vi "cornell-plot.vi"() -> ()   [LabVIEW 2020]
uses:
  cornell-Ktildesh2sides.ctl
  cursor action.ctl
  2Dwindow.ctl
  array action.ctl
  16981a69-1a1c-c642-ac20-7ef28ecb8088.vi
  replace cursor action stack.vi
  Q -- range multiplier -- real -- V2.vi
  Q - not nan and gtr than zero - Real.vi
  Q - not nan -- real.vi
  Q -- check range -- i -- real.vi
  array - smart min max.vi
  cornell-K0edges.vi
  cornell-K0s.vi
  <vilib>/Comparison/Less/Less Functor/Less Functor.lvclass
panel:
  in  "everything I need to know about heat conductivity and I mean everything":T1(tab)
  in  "parameter selectors":enum32{"Page 1"}(tab)
  in  "scale gauge: Plot: complex plane":dbl(slide)=6.232708 min=0.0 max=0.3 step=1e-06 scale=0.01..100000.0 scale format="%#_3p"
  out "Plot: sweep window":cluster{"Freq out (Hz)":dbl[], dbl[]}[](graph)
  out "Ktilde":cdb=0.005910268621655171+0.3162087805454639i format="%#_2p"
  in  "what to plot":T2=enum."plot: two½"
  in  "ω0 (rad/sec)":dbl(slide)=6.660846290809155 scale=0.001..10000.0 scale format="%#_2p"
  in  "parameter selectors 3":enum32{"Page 1"}(tab)
  out "Plot: vs s":cluster{dbl[], dbl[]}[](graph)
  in  "scale gauge: Plot: vs s":dbl(slide)=0.5231559999999998 min=0.0 max=0.3 step=1e-06 scale=0.01..10.0 scale format="%#_3p"
  in  "sample pars":T3={"τR (sec)"=0.154639, "L2DS (sec)"=3.81679389313, "τL (sec)"=10.0, "s/L"=0.0, "h/L"=0.22900799999999996} {"h/L" min=0.0 max=0.3 step=1e-06 scale=0.0..1.0 scale format="%#_3p"; "s/L" min=0.0 max=0.3 step=1e-06 scale=0.0..1.0 scale format="%#_3p"; "τL (sec)" min=0.0 max=0.3 step=1e-06 scale=0.0..100.0 scale format="%#_3p"; "L2DS (sec)" min=0.0 max=0.3 step=1e-12 scale=0.001..10.0 scale format="%#_3p"; "τR (sec)" min=0.0 max=0.3 step=1e-06 scale=0.0..100.0 scale format="%#_3p"}
  in  "plot pars":T4={"# of terms in the series"=500, "# plot points"=738, "min ω (rad/sec)"=0.0009999999999999994, "max ω (rad/sec)"=10000.00000000001} {"max ω (rad/sec)" scale=0.001..5000.0; "min ω (rad/sec)" scale=0.001..5000.0; "# plot points" scale=0.001..1500.0; "# of terms in the series" scale=0.001..1000.0}
  in  "cal pars":T5={"τS (sec)"=0.611076335878, "τC (sec)"=0.039129770992, " ζ"=0.818625954198, "κ0"=1.0} {"κ0" min=0.0 max=0.3 step=1e-12 scale=1e-10..1e-07 scale format="%#_3p"; "ζ" min=0.0 max=0.3 step=1e-12 scale=0.01..1.0 scale format="%#_3p"; "τC (sec)" min=0.0 max=0.3 step=1e-12 scale=0.001..1.0 scale format="%#_3p"; "τS (sec)" min=0.0 max=0.3 step=1e-12 scale=0.001..1.0 scale format="%#_3p"}
  in  "pause!":bool
  in  "go!":bool
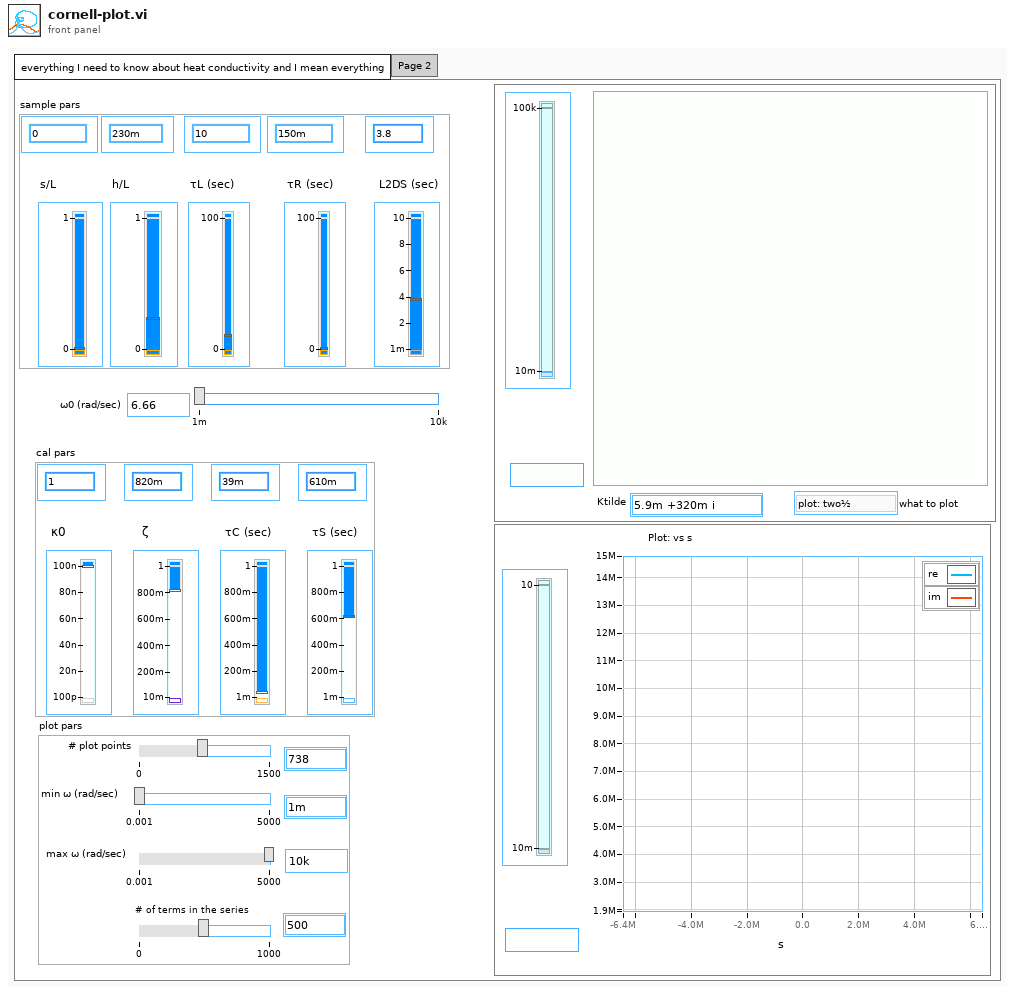
[diagram p1: front panel]
types:
  T1 = enum32{"everything I need to know about heat conductivity and I mean everything", "Page 2"}
  T2 = typedef "cornell-Ktildesh2sides.ctl" = enum16{"plot: check1", "plot: check2", "plot: one½", "plot: two½", "plot: uni½", "calc: zcoth(z)", "calc: z/sinh(z)", "calc: brute", "calc: integra", "void", "plot: nano"}
  T3 = cluster{"τR (sec)":dbl, "L2DS (sec)":dbl, "τL (sec)":dbl, "s/L":dbl, "h/L":dbl}
  T4 = cluster{"# of terms in the series":i64, "# plot points":i64, "min ω (rad/sec)":dbl, "max ω (rad/sec)":dbl}
  T5 = cluster{"τS (sec)":dbl, "τC (sec)":dbl, " ζ":dbl, "κ0":dbl}
  T6 = typedef "2Dwindow.ctl" = cluster{"window y":dbl, "center x":dbl, "center y":dbl, "window x":dbl}
  T7 = typedef "cursor action.ctl" = enum16{"range", "read", "write", "check", "zoom out", "smart zoom out", "zoom to aspect ratio 1", "zoom to win", "zoom out 20%", "zoom in 20%", "-empty", "smart zoom out&aspect", "move range left 20%", "move range right 20%", "move range up 20%", "move range down 20%", "zoom to X win", "zoom to Y win", "zoom out X", "zoom out Y", "zoom in X", "zoom in Y", "check plot scale", "set plot color", "set Xlabel", "set Ylabel", "set cursor color"}
  T8 = typedef "array action.ctl" = enum16{"generate range", "generate log range"}
  T9 = typedef "eventvkey.ctl" = enum16{"ASCII", "Enter", "Return", "Shift", "Ctrl", "Alt", "Cmd", "Opt", "Caps", "NumLock", "Clear", "Break", "Up", "Down", "Left", "Right", "Insert", "Delete", "Home", "End", "PageUp", "PageDown", "Escape", "Help", "Pause", "ScrollLock", "F1", "F2", "F3", "F4", "F5", "F6", "F7", "F8", "F9", "F10", "F11", "F12", "F13", "F14", "F15", "F16", "F17", "F18", "F19", "F20", "F21", "F22", "F23", "F24", "Play", "VolumeUp", "VolumeDown", "Mute", "Two Byte Char"}
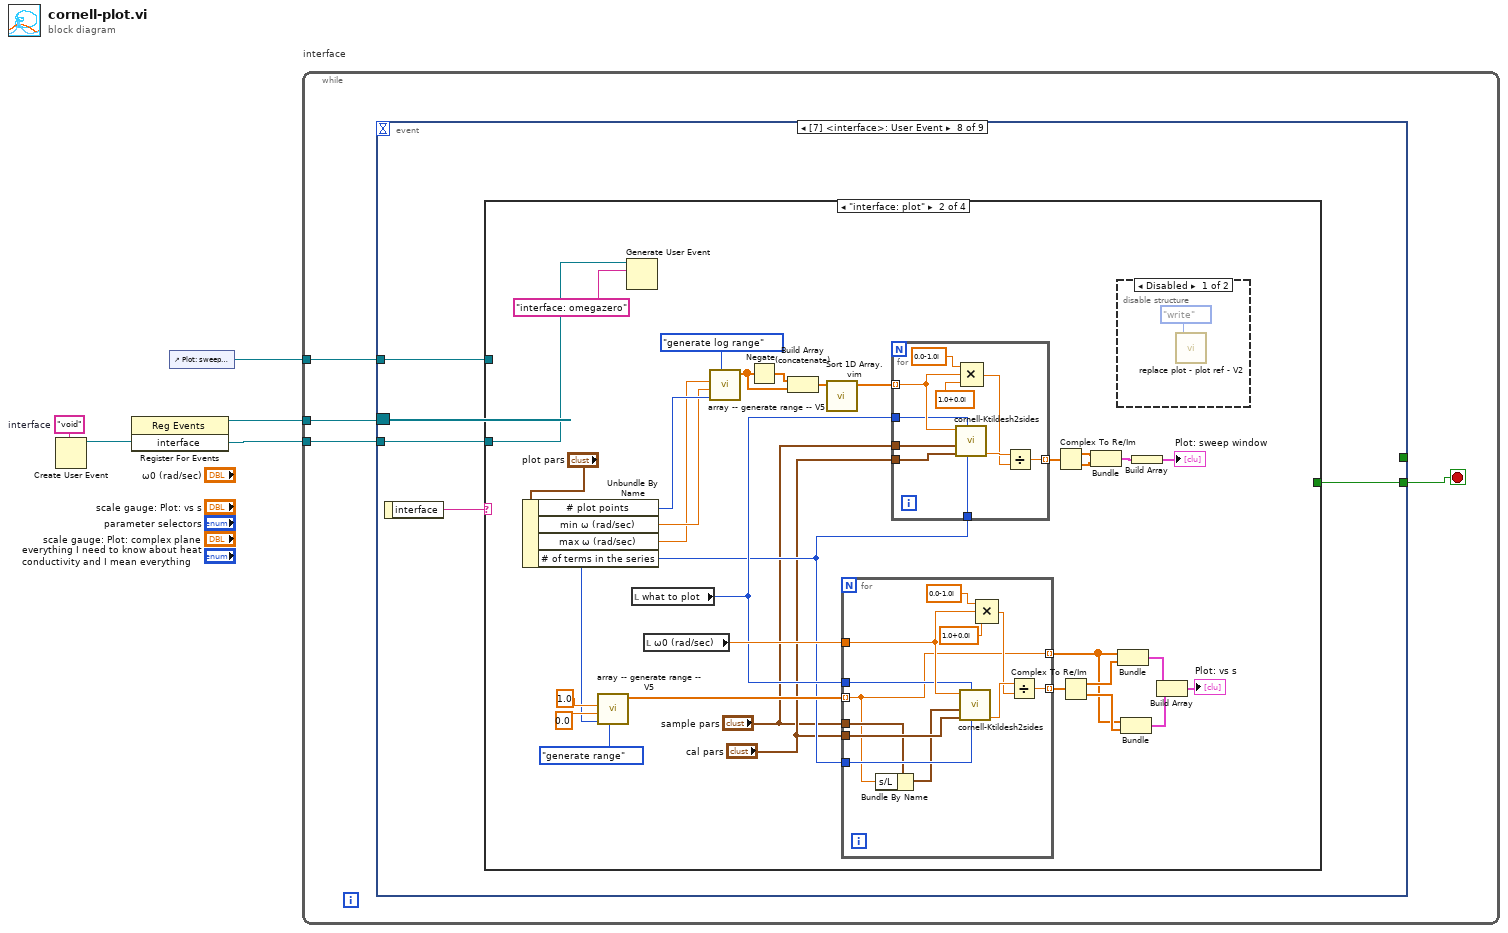
[diagram p0: block diagram]
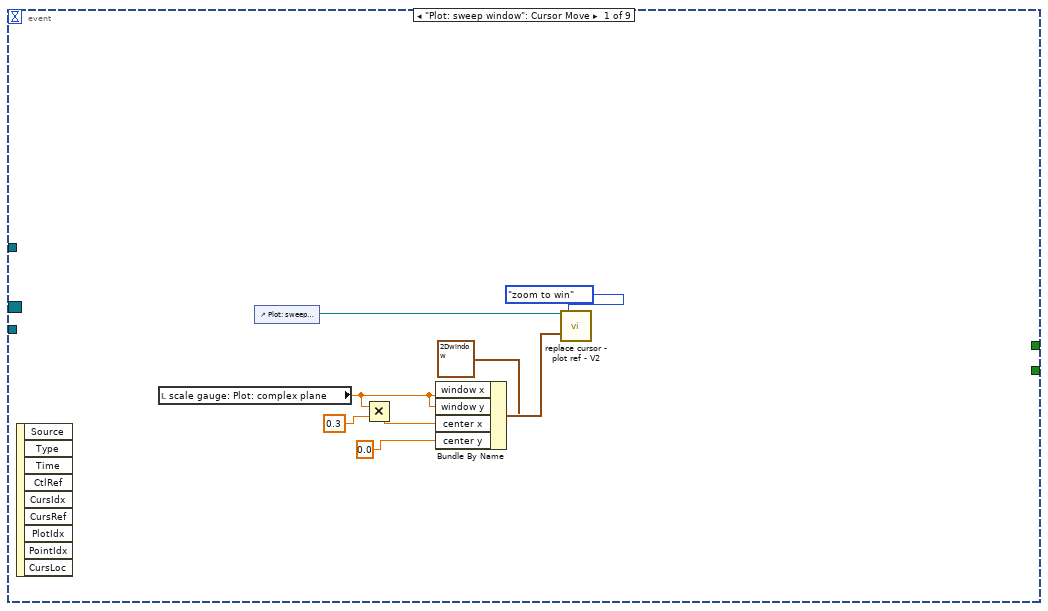
[diagram p2: hidden frame]
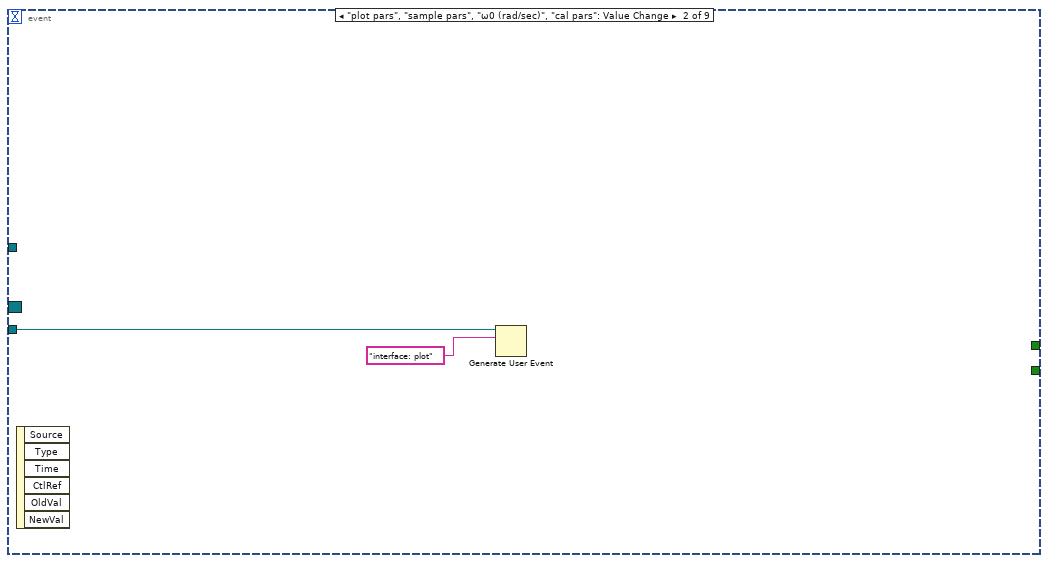
[diagram p3: hidden frame]
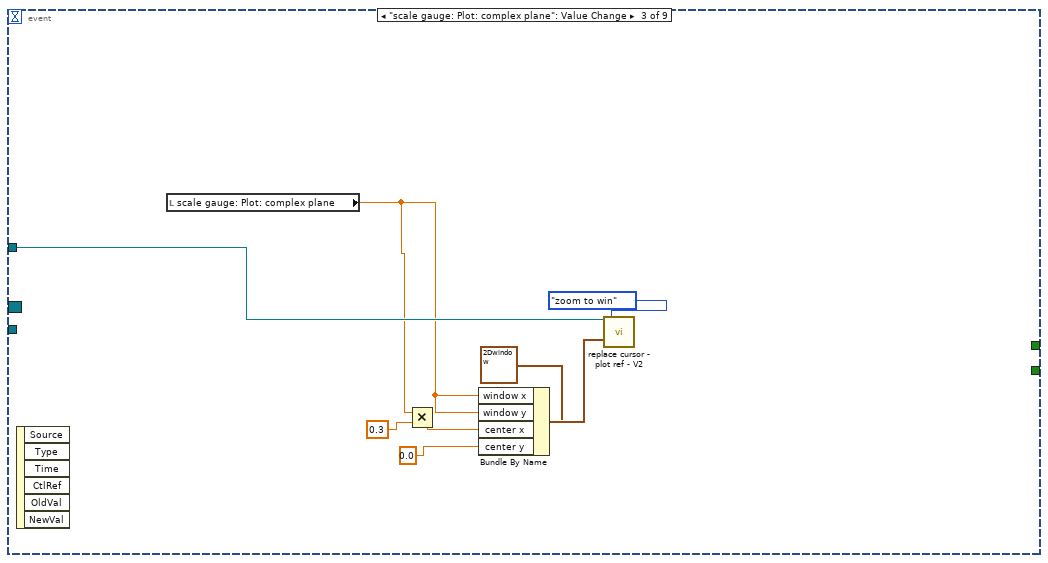
[diagram p4: hidden frame]
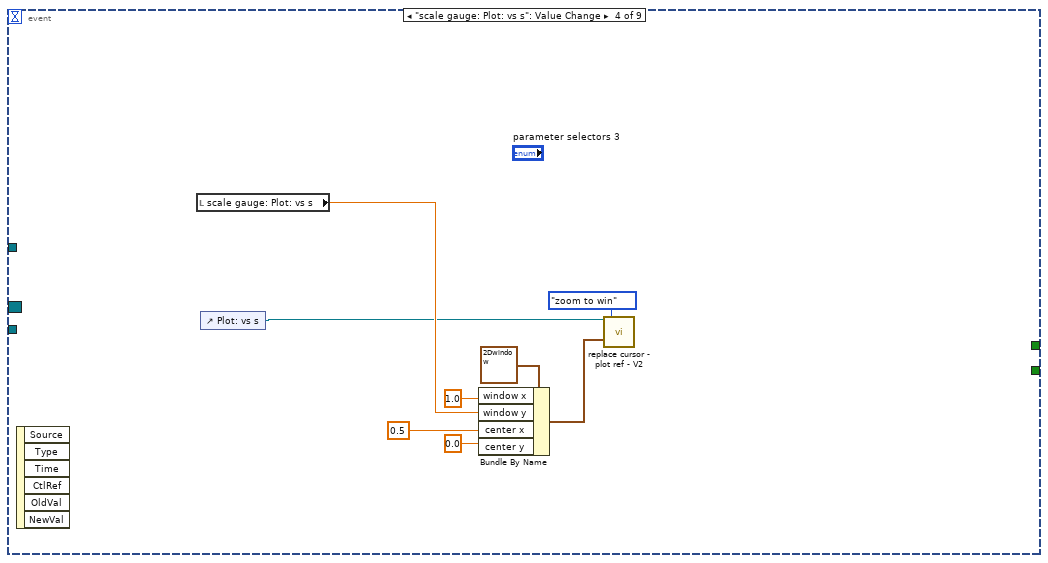
[diagram p5: hidden frame]
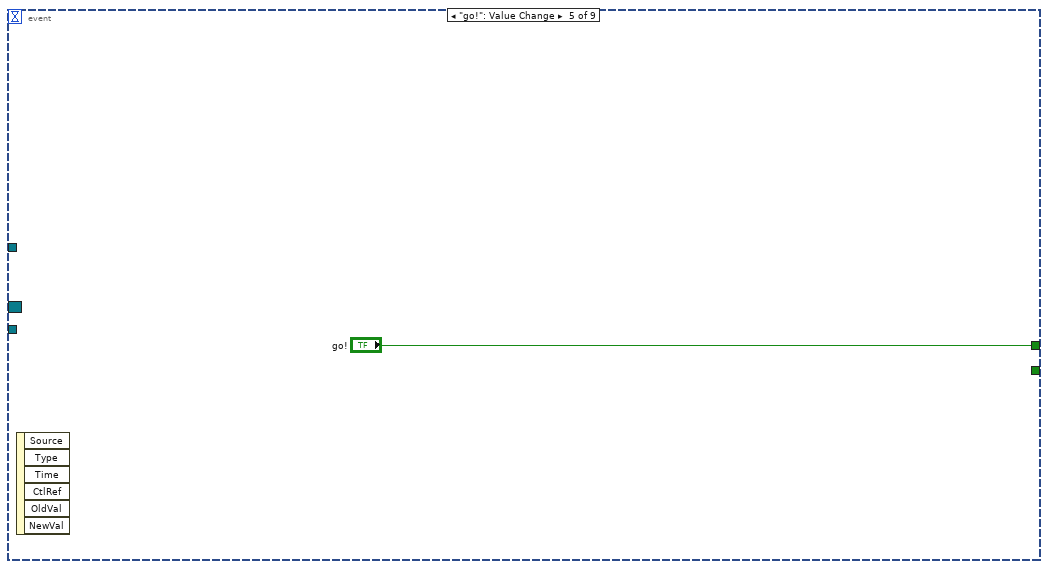
[diagram p6: hidden frame]
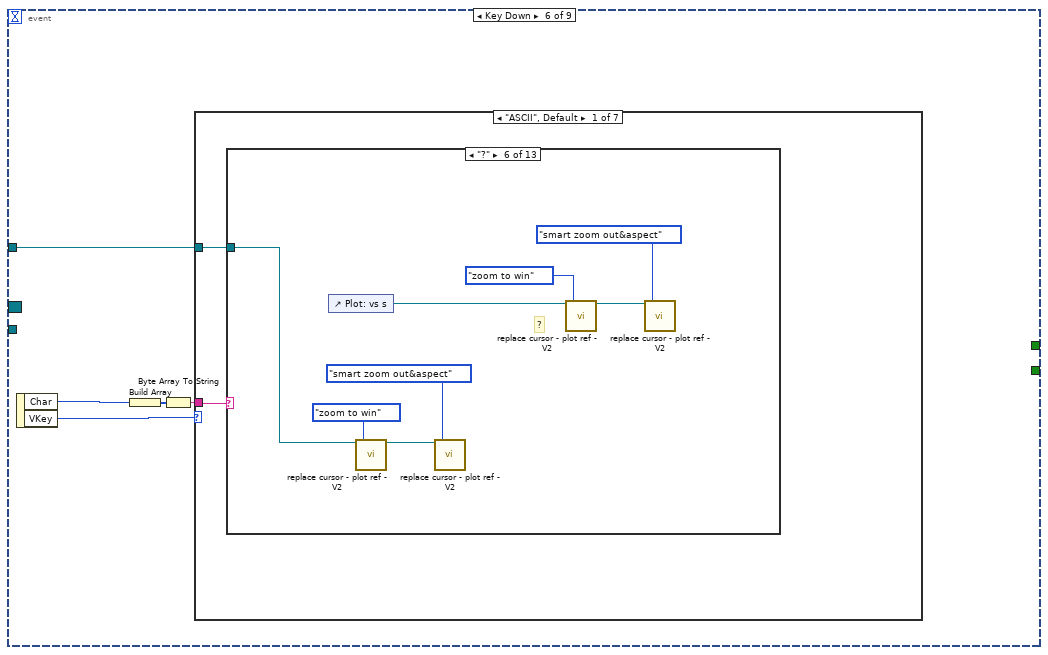
[diagram p7: hidden frame]
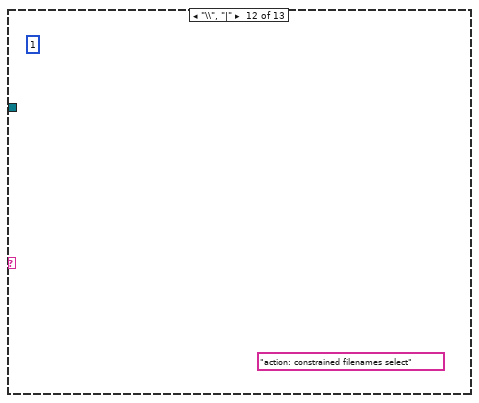
[diagram p18: hidden frame]
diagram:
  w3 = "void"  # interface
  n1 = Create User Event(user event datatype=w3) -> (user event=w1:refnum<user-event>)  [unwired: 1 in, 1 out]
  n2 = register-events(w1) -> (reference out=w4:refnum<event-registration>)  [unwired: 2 in, 1 out]
  n3 = control-ref of="Plot: sweep window"() -> (w2:refnum<vi>)
  n4 = while "interface" {
    tunnel: w4 -> [w8]
    tunnel: w2 -> [w7]
    tunnel: w1 -> [w6]
    stop <- w5 stop-if-true
    n5 = event shown="[7] <interface>: User Event" {
      selector: w8 -> [_ _ _ _ _ _ _ _ _]
      dyn-events: _ -> [_ _ _ _ _ _ _ _ _]
      timeout: _ -> [_ _ _ _ _ _ _ _ _]
      tunnel: [_ _ _ _ "go!" _ "pause!" _ _] -> _
      tunnel: w7 -> [_ _ w20 _ _ w36 _ w60 _]
      tunnel: w6 -> [_ w17 _ _ _ _ _ w59 w138]
      tunnel: [_ _ _ _ _ _ _ w61 _] -> w5
      event "Plot: sweep window": Cursor Move {
        n6 = event-data() -> ()  [unwired: 1 in, 9 out]
        n7 = local read "scale gauge: Plot: complex plane"() -> (w15:dbl)
        n8 = control-ref of="Plot: sweep window"() -> (w14:refnum<vi>)
        n9 = Multiply(x=w15, y=0.3) -> (x*y=w16:dbl)
        n10 = Bundle By Name(cluster=T6 {"window y"=0.0021014740628288917, "center x"=44850.89441339177, "center y"=2.5658109925320947, "window x"=17480.201988350764} ("window IN"), "window x"=w15, "window y"=w15, "center x"=w16, "center y"=0.0) -> (w13:T6)
        n11 = call "replace cursor - plot ref - V2.vi"("Plot ref in"=w14, "window IN"=w13, "cursor action"=cursor_action."zoom to win") -> ()  [unwired: 13 in, 4 out]
      }
      event "plot pars", "sample pars", "ω0 (rad/sec)", "cal pars": Value Change {
        n12 = event-data() -> ()  [unwired: 1 in, 6 out]
        n13 = Generate User Event(user event=w17, event data cluster="interface: plot" ("event data")) -> ()  [unwired: 2 in, 2 out]
      }
      event "scale gauge: Plot: complex plane": Value Change {
        n14 = event-data() -> ()  [unwired: 1 in, 6 out]
        n15 = local read "scale gauge: Plot: complex plane"() -> (w19:dbl)
        n16 = Multiply(x=w19, y=0.3) -> (x*y=w26:dbl)
        n17 = Bundle By Name(cluster=T6 {"window y"=0.0021014740628288917, "center x"=44850.89441339177, "center y"=2.5658109925320947, "window x"=17480.201988350764} ("window IN"), "window x"=w19, "window y"=w19, "center x"=w26, "center y"=0.0) -> (w25:T6)
        n18 = call "replace cursor - plot ref - V2.vi"("Plot ref in"=w20, "window IN"=w25, "cursor action"=cursor_action."zoom to win") -> ()  [unwired: 13 in, 4 out]
      }
      event "scale gauge: Plot: vs s": Value Change {
        n19 = event-data() -> ()  [unwired: 1 in, 6 out]
        n20 = local read "scale gauge: Plot: vs s"() -> (w30:dbl)
        n21 = control-ref of="Plot: vs s"() -> (w29:refnum<vi>)
        n22 = Bundle By Name(cluster=T6 {"window y"=0.0021014740628288917, "center x"=44850.89441339177, "center y"=2.5658109925320947, "window x"=17480.201988350764} ("window IN"), "window x"=1.0, "window y"=w30, "center x"=0.5, "center y"=0.0) -> (w34:T6)
        n23 = call "replace cursor - plot ref - V2.vi"("Plot ref in"=w29, "window IN"=w34, "cursor action"=cursor_action."zoom to win") -> ()  [unwired: 13 in, 4 out]
      }
      event "go!": Value Change {
        n24 = event-data() -> ()  [unwired: 1 in, 6 out]
      }
      event Key Down {
        n25 = event-data() -> ("Char"=w38:i16, "VKey"=w40:T9)  [unwired: 1 in]
        n26 = Build Array(w38) -> (w39:i16[])
        n27 = Byte Array To String(unsigned byte array=w39) -> (string=w37:string)
        n28 = case shown="\"ASCII\", Default" w40 {
          selector: w40 -> [_ _ _ _ _ _ w52]
          tunnel: w37 -> [w42 _ _ _ _ _ _]
          tunnel: w36 -> [w41 _ _ _ _ _ w51]
          frame "ASCII", Default {
            n29 = case shown="\"?\"" w42 {
              tunnel: w41 -> [_ _ _ _ _ w47 _ _ _ _ _ _ _]
              frame "0", Default {
              }
              frame "a" {
              }
              frame "s" {
              }
              frame "l" {
              }
              frame " " {
              }
              frame "?" {
                # "?"
                n30 = control-ref of="Plot: vs s"() -> (w43:refnum<vi>)
                n31 = call "replace cursor - plot ref - V2.vi"("Plot ref in"=w47, "cursor action"=cursor_action."zoom to win") -> ("Plot ref out"=w50:refnum<vi>)  [unwired: 14 in, 3 out]
                n32 = call "replace cursor - plot ref - V2.vi"("Plot ref in"=w50, "cursor action"=cursor_action."smart zoom out&aspect") -> ()  [unwired: 14 in, 4 out]
                n33 = call "replace cursor - plot ref - V2.vi"("Plot ref in"=w43, "cursor action"=cursor_action."zoom to win") -> ("Plot ref out"=w46:refnum<vi>)  [unwired: 14 in, 3 out]
                n34 = call "replace cursor - plot ref - V2.vi"("Plot ref in"=w46, "cursor action"=cursor_action."smart zoom out&aspect") -> ()  [unwired: 14 in, 4 out]
              }
              frame "+", ",", "-", ".", "<", "=", ">" {
              }
              frame "b" {
              }
              frame "u" {
              }
              frame "p" {
              }
              frame "q" {
              }
              frame "\\", "|" {
                (unwired) 1
                (unwired) "action: constrained filenames select" ("event data")
              }
              frame "m" {
              }
            }
          }
          frame "Escape" {
          }
          frame "PageUp" {
          }
          frame "Enter" {
          }
          frame "Caps" {
          }
          frame "PageDown" {
          }
          frame "Up".."Right" {
            n35 = case shown="\"Down\"" w52 {
              tunnel: [cursor_action."zoom in 20%" ("cursor action") cursor_action."zoom out 20%" ("cursor action") cursor_action."zoom out 20%" ("cursor action") cursor_action."zoom in 20%" ("cursor action")] -> w53
              frame "Up", Default {
              }
              frame "Down" {
              }
              frame "Left" {
              }
              frame "Right" {
              }
            }
            n36 = call "replace cursor - plot ref - V2.vi"("Plot ref in"=w51, "cursor action"=w53) -> ()  [unwired: 14 in, 4 out]
          }
        }
      }
      event "pause!": Value Change {
        n37 = event-data() -> ()  [unwired: 1 in, 6 out]
      }
      event User Event {
        n38 = event-data() -> ("interface"=w62:string)  [unwired: 1 in]
        n39 = case shown="\"interface: plot\"" w62 {
          tunnel: [_ _ TRUE _] -> w61
          tunnel: w60 -> [_ _ _ w130]
          tunnel: w59 -> [_ w84 _ _]
          frame "void", Default {
          }
          frame "interface: plot" {
            n40 = Unbundle By Name("plot pars") -> ("# plot points"=w69:i64, "min ω (rad/sec)"=w67:dbl, "max ω (rad/sec)"=w66:dbl, "# of terms in the series"=w68:i64)
            n41 = call "array -- generate range -- V5.vi"("action"=array_action."generate range", "ω points"=w69, "ω from"=0.0, "ω to"=1.0) -> ("ω out"=w71:dbl[])  [unwired: 7 in]
            n42 = Generate User Event(user event=w84, event data cluster="interface: omegazero" ("event data")) -> ()  [unwired: 2 in, 2 out]
            n43 = local read "what to plot"() -> (w70:T2)
            n44 = local read "ω0 (rad/sec)"() -> (w79:dbl)
            n45 = call "array -- generate range -- V5.vi"("action"=array_action."generate log range", "ω points"=w69, "ω from"=w67, "ω to"=w66) -> ("ω out"=w87:dbl[])  [unwired: 7 in]
            n46 = Negate(x=w87) -> (-x=w88:dbl[])
            n47 = Build Array (concatenate)(w88, w87) -> (w86:dbl[])
            n48 = call "Sort 1D Array.vim"("unsorted array"=w86) -> ("sorted array"=w83:dbl[])  [unwired: 10 in]
            n49 = for {
              tunnel: w71 -> [w95] mode=indexing
              tunnel: [w105] -> w76 mode=indexing
              tunnel: w68 -> [w104]
              tunnel: w79 -> [w100]
              tunnel: [w95] -> w73 mode=indexing
              tunnel: w70 -> [w99]
              tunnel: "cal pars" -> [w98]
              tunnel: "sample pars" -> [w97]
              n50 = Bundle By Name(cluster=w97, "s/L"=w95) -> (w96:T3)
              n51 = call "cornell-Ktildesh2sides.vi"("#of terms"=w104, "action"=w99, "cal pars"=w98, "sample pars"=w96, "ω"=w100) -> ("Ks(ω)"=w106:cdb)  [unwired: 5 in]
              n52 = Compound Arithmetic op=MULTIPLY(cdb 0.0-1.0i, w100, cdb 1.0+0.0i) -> (w102:cdb)
              n53 = Divide(x=w106, y=w102) -> (x/y=w105:cdb)
            }
            n54 = for {
              tunnel: w83 -> [w114] mode=indexing
              tunnel: [w117] -> w93 mode=indexing
              tunnel: w68 -> [w116]
              tunnel: w70 -> [w111]
              tunnel: "cal pars" -> [w110]
              tunnel: "sample pars" -> [w109]
              n55 = call "cornell-Ktildesh2sides.vi"("#of terms"=w116, "action"=w111, "cal pars"=w110, "sample pars"=w109, "ω"=w114) -> ("Ks(ω)"=w118:cdb)  [unwired: 5 in]
              n56 = Compound Arithmetic op=MULTIPLY(cdb 0.0-1.0i, w114, cdb 1.0+0.0i) -> (w113:cdb)
              n57 = Divide(x=w118, y=w113) -> (x/y=w117:cdb)
            }
            n58 = Complex To Re/Im(x + iy=w93) -> (x=w92:dbl[], y=w91:dbl[])
            n59 = Complex To Re/Im(x + iy=w76) -> (x=w75:dbl[], y=w74:dbl[])
            n60 = Bundle(w92, w91) -> (w90:cluster{dbl[], dbl[]})  [unwired: 1 in]
            n61 = disable-structure shown="Disabled" {
              frame Disabled {
                n62 = call "replace plot - plot ref - V2.vi"("cursor action"=cursor_action."write") -> ("Array X IN"=w108:dbl[])  [unwired: 14 in, 4 out]
              }
              frame Enabled {
              }
            }
            n63 = Bundle(w73, w75) -> (w78:cluster{dbl[], dbl[]})  [unwired: 1 in]
            n64 = Bundle(w73, w74) -> (w72:cluster{dbl[], dbl[]})  [unwired: 1 in]
            n65 = Build Array(w90) -> (→"Plot: sweep window":cluster{dbl[], dbl[]}[])
            n66 = Build Array(w78, w72) -> (→"Plot: vs s":cluster{dbl[], dbl[]}[])
          }
          frame "interface: exit" {
          }
          frame "interface: omegazero" {
            n67 = local read "plot pars"() -> (w121:T4)
            n68 = Unbundle By Name(w121) -> ("# of terms in the series"=w120:i64)
            n69 = local read "sample pars"() -> (w123:T3)
            n70 = local read "cal pars"() -> (w122:T5)
            n71 = local read "ω0 (rad/sec)"() -> (w127:dbl)
            n72 = local read "what to plot"() -> (w124:T2)
            n73 = call "cornell-Ktildesh2sides.vi"("#of terms"=w120, "action"=w124, "cal pars"=w122, "sample pars"=w123, "ω"=w127) -> ("Ks(ω)"=w133:cdb)  [unwired: 5 in]
            n74 = Compound Arithmetic op=MULTIPLY(cdb 1.0+0.0i, w127, cdb 0.0-1.0i) -> (w126:cdb)
            n75 = Divide(x=w133, y=w126) -> (x/y=w129:cdb)
            "Ktilde" <- w129
            n76 = Complex To Re/Im(x + iy=w129) -> (x=w134:dbl, y=w135:dbl)
            n77 = call "replace cursor - plot ref - V2.vi"("Plot ref in"=w130, "new X"=w134, "new  Y"=w135, "cursor index"=0, "cursor action"=cursor_action."write") -> ()  [unwired: 11 in, 4 out]
          }
        }
      }
      event Value Change {
        n78 = event-data() -> ("NewVal"=w137:T2)  [unwired: 1 in]
        n79 = local write "what to plot"(w137) -> ()
        n80 = Generate User Event(user event=w138, event data cluster="interface: plot" ("event data")) -> ()  [unwired: 2 in, 2 out]
      }
    }
  }
